vi "init.vi"(8 "error in":errorcluster, 10 "io configuration in":refnum<class "TBM module configuration.lvclass">, 11 "io runtime in":refnum<class "io runtime.lvclass">) -> (0 "error out":errorcluster, 1 "data allocations":T1, 2 "execution settings":T4, 3 "io runtime out":refnum<class "io runtime.lvclass">)   [LabVIEW 2015, in "io runtime.lvclass"]
doc: "Provides an interface for initializing a module at runtime. While this interface performs no operations, a child should provide an override which may open any necessary references or sessions, allocate necessary memory, and perform any final configuration validataion before providing the full configuration <b>execution data</b> to the calling process."
uses:
  io runtime.lvclass
  <vilib>/NI/Tag Bus Module Framework/module configuration/TBM module configuration.lvclass
  <vilib>/NI/Tag Bus Module Framework/runtime/execution settings.ctl
  <vilib>/NI/Tag Bus Module Framework/channel/data tables.ctl
  <vilib>/NI/Tag Bus/dictionary/data dictionary.lvclass
  <vilib>/NI/Tag Bus/dictionary table pair.ctl
  <vilib>/NI/Tag Bus/table/data table.ctl
  configuration/io configuration.lvclass
  io runtime.lvclass/io runtime.ctl
  <vilib>/NI/Tag Bus Module Framework/channel/TBM channel.lvclass
  <vilib>/NI/Tag Bus Module Framework/runtime/TBM module execution interface.lvclass
  <vilib>/NI/Tag Bus/tag bus.lvlib
  <vilib>/NI/Tag Bus/table/data table.lvlib
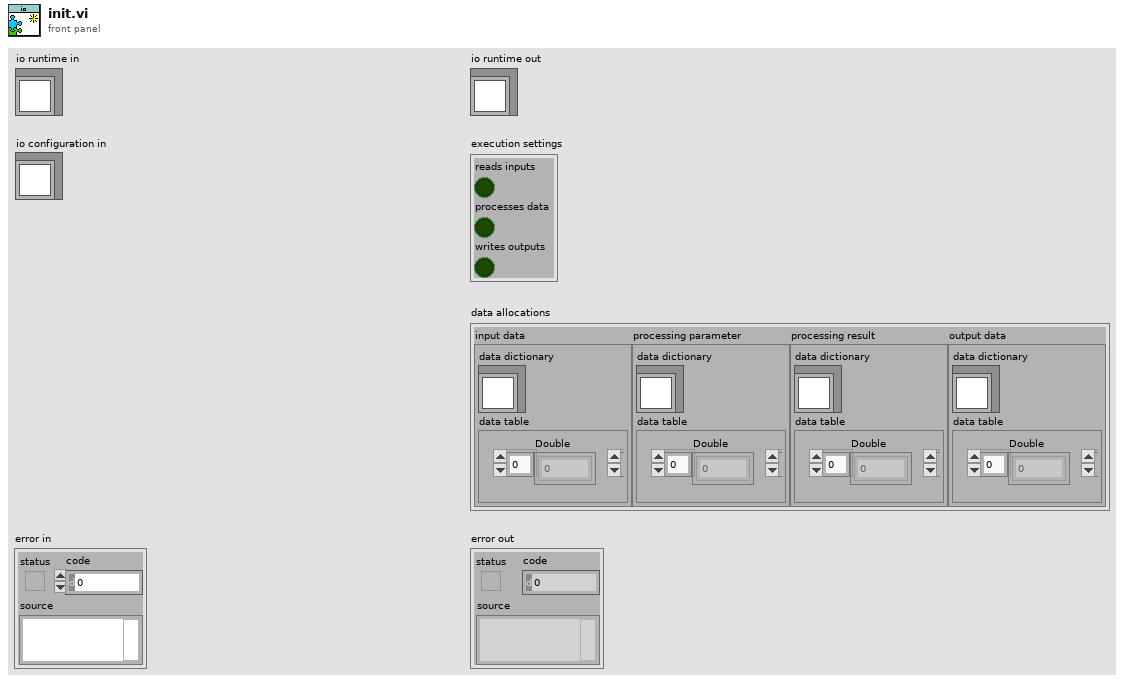
[diagram p1: front panel]
types:
  T1 = typedef "TBM channel.lvclass/data tables.ctl" = cluster{"input data":T2, "processing parameter":T2, "processing result":T2, "output data":T2}
  T2 = typedef "tag bus.lvlib/dictionary table pair.ctl" = cluster{"data dictionary":refnum<class "data dictionary.lvclass">, "data table":T3}
  T3 = typedef "tag bus.lvlib/data table.lvlib/data table.ctl" = cluster{"Double":dbl[], "Single":sgl[], "I64":i64[], "I32":i32[], "I16":i16[], "I8":i8[], "U64":u64[], "U32":u32[], "U16":u16[], "U8":u8[], "Boolean":bool[], "String":string[], "Array of Double":cluster{"DBL Array":dbl[]}[], "Array of Single":cluster{"SGL Array":sgl[]}[], "Array of I64":cluster{"I64 Array":i64[]}[], "Array of I32":cluster{"I32 Array":i32[]}[], "Array of I16":cluster{"I16 Array":i16[]}[], "Array of I8":cluster{"I8 Array":i8[]}[], "Array of U64":cluster{"U64 Array":u64[]}[], "Array of U32":cluster{"U32 Array":u32[]}[], "Array of U16":cluster{"U16 Array":u16[]}[], "Array of U8":cluster{"U8 Array":u8[]}[], "Array of Boolean":cluster{"Boolean Array":bool[]}[], "Array of String":cluster{"String Array":string[]}[]}
  T4 = typedef "TBM module execution interface.lvclass/execution settings.ctl" = cluster{"reads inputs":bool, "processes data":bool, "writes outputs":bool}
  T5 = typedef "io runtime.lvclass/control index set.ctl" = cluster{"data type":T6, "fpga res type":T7[], "fpga resource":refnum<k20>[], "data indexes":i32[], "fifo timeout":refnum<k20>[], "fifo reset":refnum<k20>[], "fifo average":i32[], "fifo samples":u32[], "fifo channels":u32[]}
  T6 = typedef "tag bus.lvlib/tag descriptor.lvclass/Data Type.ctl" = enum16{"Double", "Single", "I64", "I32", "I16", "I8", "U64", "U32", "U16", "U8", "Boolean", "String", "Array of Double", "Array of Single", "Array of I64", "Array of I32", "Array of I16", "Array of I8", "Array of U64", "Array of U32", "Array of U16", "Array of U8", "Array of Boolean", "Array of String"}
  T7 = typedef "io configuration.lvclass/fpga resource supported data types.ctl" = enum16{"Invalid Type", "Single", "I64", "I32", "I16", "I8", "U64", "U32", "U16", "U8", "Boolean", "FXP I,20,5", "FXP I,24,5", "FXP I,24,10", "Fifo 1023,I16"}
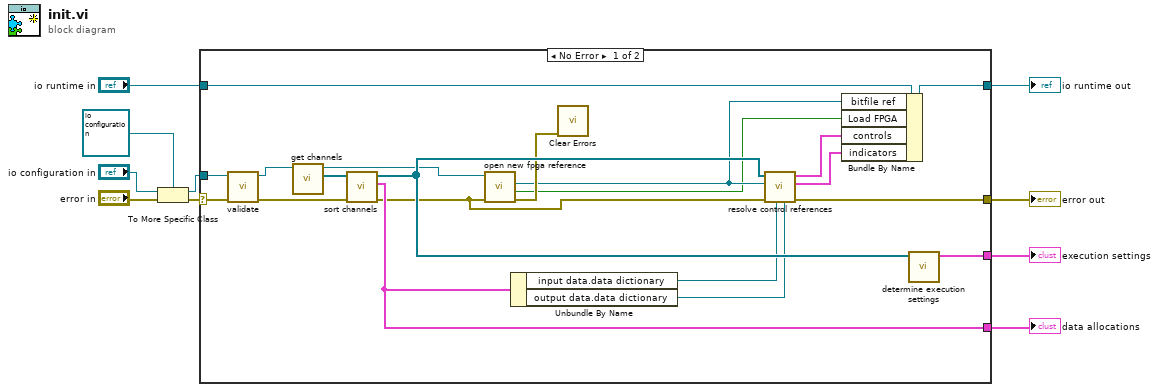
[diagram p0: block diagram]
diagram:
  n1 = To More Specific Class(target class=refnum<class "io configuration.lvclass"> refnum ("Synchronous module configuration"), reference="io configuration in", error in="error in") -> (specific class reference=w9:refnum<class "io configuration.lvclass">, error out=w10:errorcluster)
  n2 = case shown="No Error" w10 {
    selector: w10 -> [w27 w31]
    tunnel: w9 -> [w17 _]
    tunnel: "io runtime in" -> [w30 w32]
    tunnel: [w24 w32] -> w4
    tunnel: [w23 w31] -> w3
    tunnel: [w20 _] -> w1
    tunnel: [w29 _] -> w2
    frame No Error {
      n3 = call-dynamic "validate.vi"("error in"=w27, "io configuration in"=w17) -> ("error out"=w28:errorcluster, "io configuration out"=w26:refnum<class "io configuration.lvclass">)  [unwired: 8 in]
      n4 = call-dynamic "get channels.vi"("io configuration in"=w26) -> ("channels"=w25:refnum<class "TBM channel.lvclass">[], "io configuration out"=w16:refnum<class "io configuration.lvclass">)  [unwired: 9 in]
      n5 = call <vilib>:"sort channels.vi"("error in"=w28, "channels in"=w25) -> ("error out"=w14:errorcluster, "data allocations"=w20:T1, "channels out"=w21:refnum<class "TBM channel.lvclass">[])  [unwired: 7 in]
      n6 = call "open new fpga reference.vi"("error in"=w14, "io configuration in"=w16) -> ("error out"=w15:errorcluster, "Load FPGA"=w11:bool, "Bitfile reference out"=w13:refnum<k20>)  [unwired: 6 in, 1 out]
      n7 = Unbundle By Name(w20) -> ("input data.data dictionary"=w18:refnum<class "data dictionary.lvclass">, "output data.data dictionary"=w19:refnum<class "data dictionary.lvclass">)
      n8 = call <vilib>:"Clear Errors.vi"("error in (no error)"=w15) -> ()  [unwired: 5 in, 2 out]
      n9 = call "resolve control references.vi"("output dictionary"=w19, "input dictionary"=w18, "error in"=w14, "bitfile ref"=w13, "channels in"=w21) -> ("error out"=w23:errorcluster, "indicators"=w22:T5[], "controls"=w12:T5[])  [unwired: 4 in]
      n10 = Bundle By Name(cluster=w30, "bitfile ref"=w13, "Load FPGA"=w11, "controls"=w12, "indicators"=w22) -> (w24:refnum<class "io runtime.lvclass">)
      n11 = call <vilib>:"determine execution settings.vi"("channels"=w21) -> ("execution settings"=w29:T4)  [unwired: 10 in]
    }
    frame Error {
    }
  }
  "error out" <- w3
  "io runtime out" <- w4
  "execution settings" <- w2
  "data allocations" <- w1
